vi "Reset.vi"(8 "error in (no error)":errorcluster, 10 "Context in":refnum<class "Context.lvclass">, 11 "Timed Out in":refnum<class "Timed Out.lvclass">) -> (0 "error out":errorcluster, 2 "Context out":refnum<class "Context.lvclass">, 3 "State out":refnum<class "State.lvclass">)   [LabVIEW 2024, in "State.lvlib" / "Timed Out.lvclass"]
uses:
  State/State.lvclass
  Context/Context/Context.lvclass
  Timed Out.lvclass
  Timed Out.lvclass/Timed Out.ctl
  Idle/Idle.lvclass
  C:/Users/uspoaotto/OneDrive - Oregon Tool/Desktop/working copies/stateMachineActor/src/State Machine/State/Container State/Container State.lvclass
  C:/Users/uspoaotto/OneDrive - Oregon Tool/Desktop/working copies/stateMachineActor/src/State Machine/State/State/State.lvclass
  C:/Users/uspoaotto/OneDrive - Oregon Tool/Desktop/working copies/stateMachineActor/src/State Machine/State/Timed Out/Timed Out.lvclass
  C:/Users/uspoaotto/OneDrive - Oregon Tool/Desktop/working copies/stateMachineActor/src/State Machine/State/Idle/Idle.lvclass
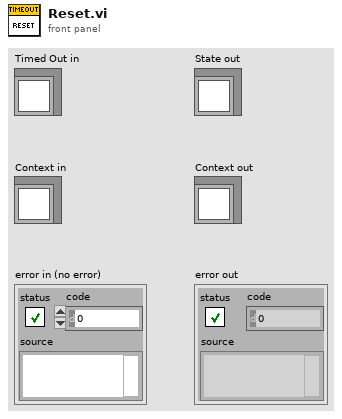
[diagram p1: front panel]
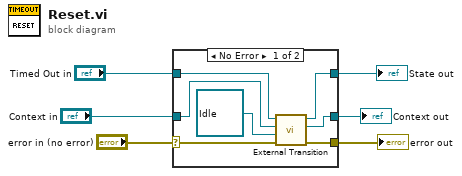
[diagram p0: block diagram]
diagram:
  n1 = case shown="No Error" "error in (no error)" {
    selector: "error in (no error)" -> [w12 w14]
    tunnel: "Context in" -> [w11 w15]
    tunnel: "Timed Out in" -> [w10 w16]
    tunnel: [w9 w16] -> w3
    tunnel: [w8 w15] -> w2
    tunnel: [w7 w14] -> w1
    frame No Error {
      n2 = call "External Transition.vi"("error in (no error)"=w12, "Target"=refnum<class "Idle.lvclass"> refnum ("State.lvlib:Idle.lvclass"), "Context in"=w11, "Source"=w10) -> ("error out"=w7:errorcluster, "Context out"=w8:refnum<class "Context.lvclass">, "State out"=w9:refnum<class "State.lvclass">)  [unwired: 5 in]
    }
    frame Error {
    }
  }
  "error out" <- w1
  "State out" <- w3
  "Context out" <- w2
